vi "通道设置.vi"(0 "Channel (0: Channel 1)":u16(ring) items=["Channel 1", "Channel 2", "Channel 3", "Channel 4", "Math", "Reference 1", "Reference 2", "Reference 3", "Reference 4", "Bus 1", "Bus 2"], 1 "范围 (10.0 V)":dbl=10.0, 2 "VISA resource name":refnum<visa-resource-name>, 3 "带宽 (0: FULL)":u16(ring) items=["FULL", "250 MHz", "150 MHz", "20 MHz"], 5 "偏置 (0.0 V)":dbl, 9 "衰减 (1)":dbl=1.0, 11 "耦合(1: DC)":u16(ring)=1 items=["AC", "DC", "Ground"], 12 "输入阻抗 (0: 1M ohm)":u16(ring) items=["1M", "75", "50"], 13 "error in (no error)":errorcluster, 14 "通道使能 (T: Enable)":bool=TRUE) -> (4 "VISA resource name out":refnum<visa-resource-name>, 15 "error out":errorcluster)   [LabVIEW 2018]
uses:
  Tektronix DPO MSO 2000 4000 Series/Tektronix DPO MSO 2000 4000 Series.lvlib
panel:
  out "写入缓冲区":string
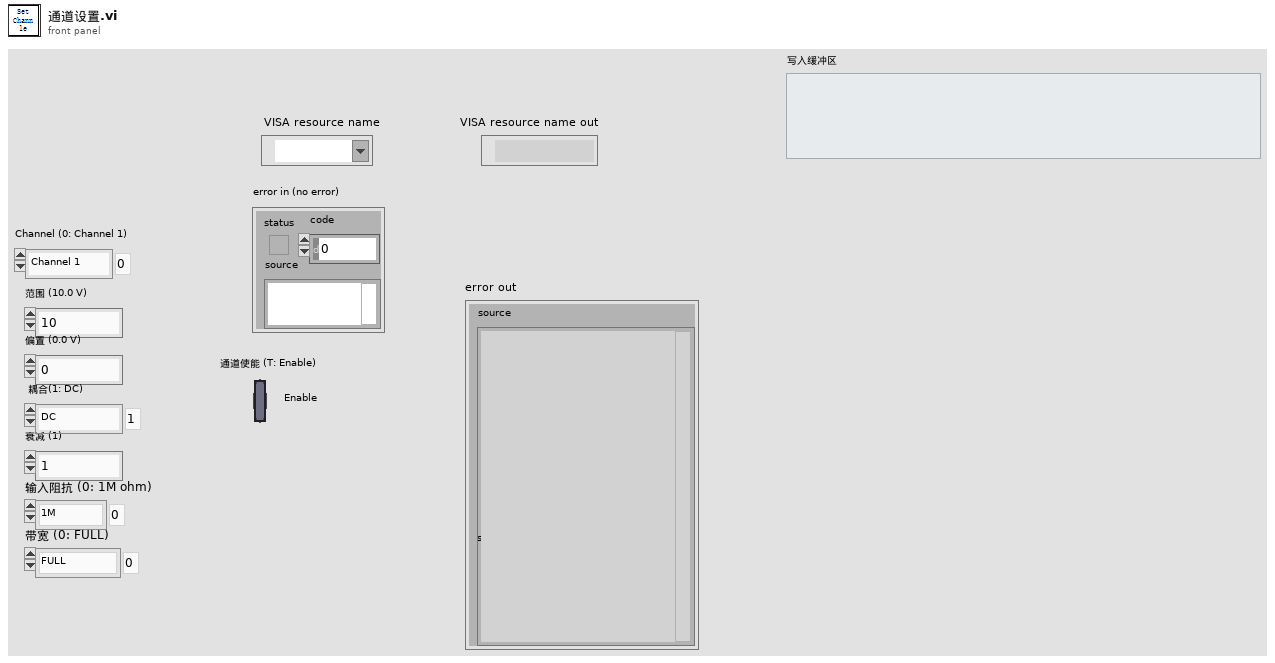
[diagram p1: front panel]
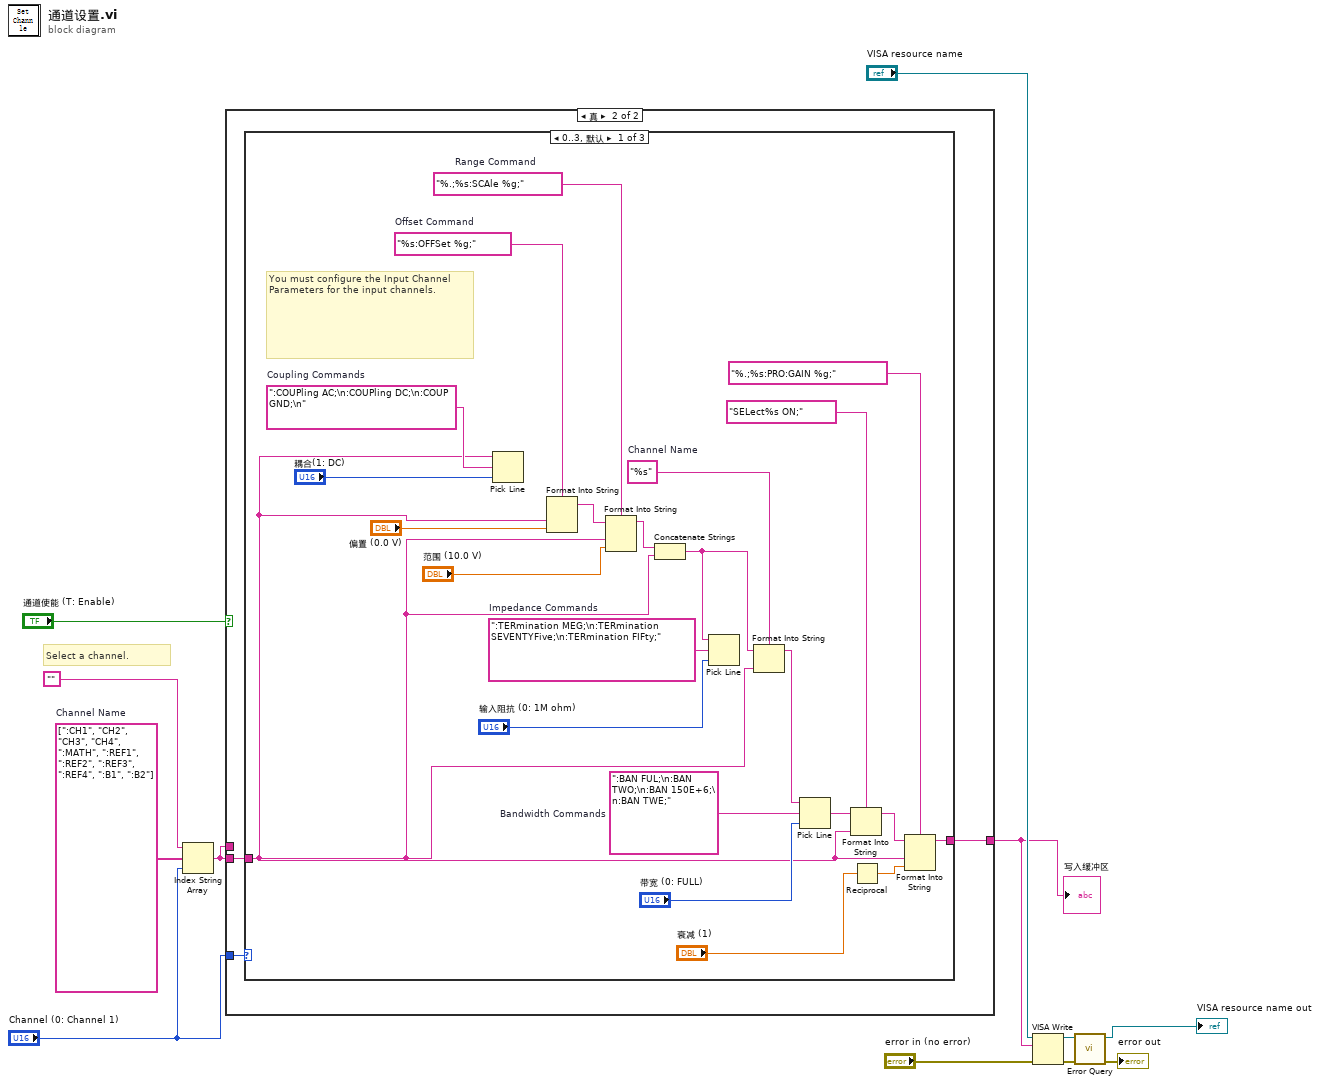
[diagram p0: block diagram]
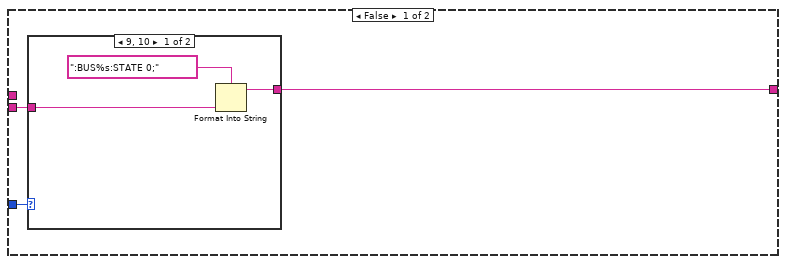
[diagram p2: hidden frame]
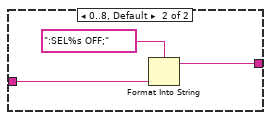
[diagram p3: hidden frame]
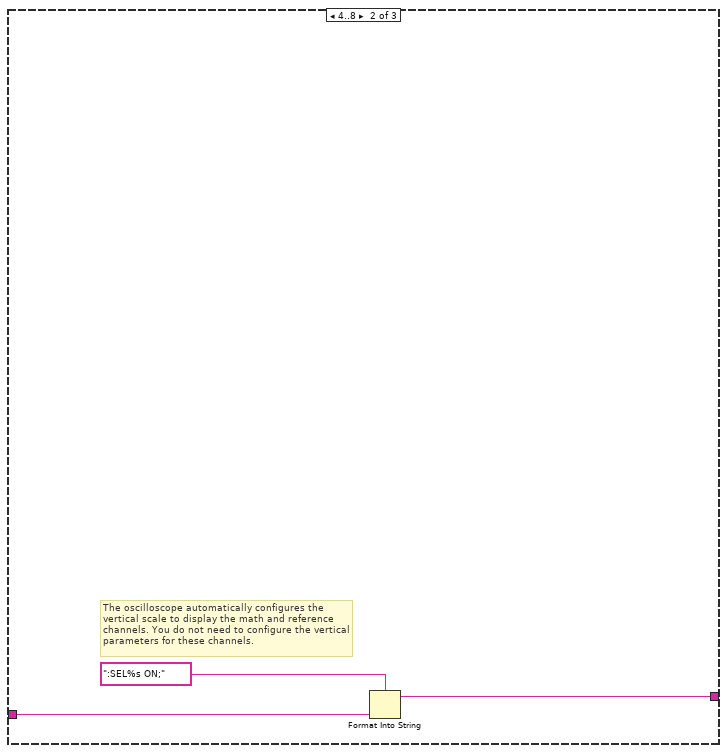
[diagram p4: hidden frame]
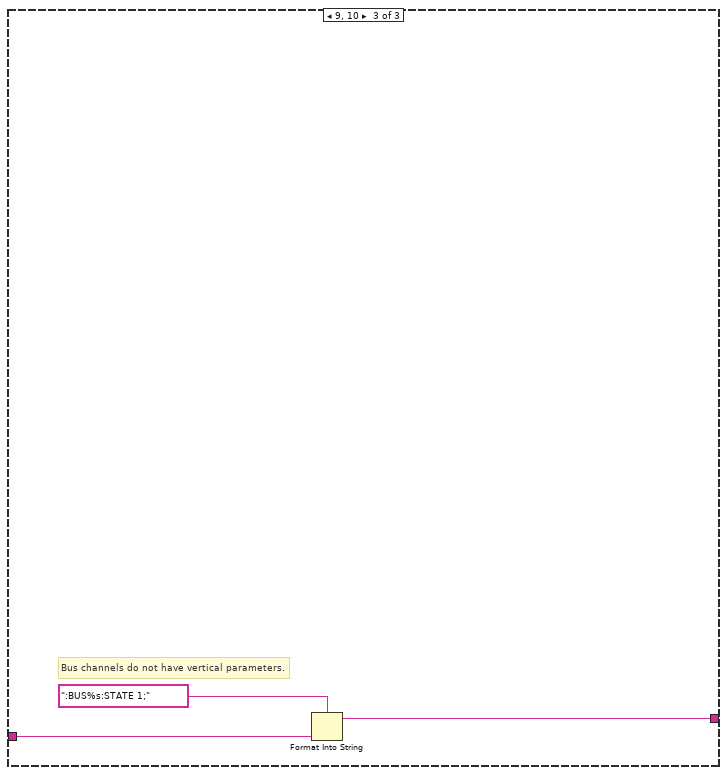
[diagram p5: hidden frame]
diagram:
  w11 = string[] [":CH1", "CH2", "CH3", "CH4", ":MATH", ":REF1", ":REF2", ":REF3", ":REF4", ":B1", ":B2"]  # Channel Name
  # "Select a channel."
  n1 = Index String Array(1:"Channel (0: Channel 1)", 2:w11, 3:"") -> (0:w8:string)
  n2 = case shown="真" "通道使能 (T: Enable)" {
    tunnel: "Channel (0: Channel 1)" -> [w15 w24]
    tunnel: [w14 w23] -> w1
    tunnel: w8 -> [_ _]
    tunnel: w8 -> [w13 w22]
    frame False {
      n3 = case shown="9, 10" w15 {
        tunnel: [w17 w20] -> w14
        tunnel: w13 -> [w16 w19]
        frame 9, 10 {
          n4 = Format Into String(format string=":BUS%s:STATE 0;", w16) -> (resulting string=w17:string)  [unwired: 2 in, 1 out]
        }
        frame 0..8, Default {
          n5 = Format Into String(format string=":SEL%s OFF;", w19) -> (resulting string=w20:string)  [unwired: 2 in, 1 out]
        }
      }
    }
    frame True {
      n6 = case shown="0..3, 默认" w24 {
        tunnel: [w31 w49 w52] -> w23
        tunnel: w22 -> [w26 w48 w51]
        frame 0..3, Default {
          w37 = ":BAN FUL;\n:BAN TWO;\n:BAN 150E+6;\n:BAN TWE;"  # Bandwidth Commands
          w39 = "%s"  # Channel Name
          w40 = ":TERmination MEG;\n:TERmination SEVENTYFive;\n:TERmination FIFty;"  # Impedance Commands
          w43 = "%.;%s:SCAle %g;"  # Range Command
          w45 = "%s:OFFSet %g;"  # Offset Command
          w47 = ":COUPling AC;\n:COUPling DC;\n:COUP GND;\n"  # Coupling Commands
          # "You must configure the Input Channel\nParameters for the input channels."
          n7 = Pick Line(string ("")=w26, multi-line string=w47, line index="耦合(1: DC)") -> ()  [unwired: 1 out]
          n8 = Format Into String(format string=w45, w26, "偏置 (0.0 V)") -> (resulting string=w42:string)  [unwired: 2 in, 1 out]
          n9 = Format Into String(format string=w43, initial string=w42, w26, "范围 (10.0 V)") -> (resulting string=w27:string)  [unwired: 1 in, 1 out]
          n10 = Concatenate Strings(w27, w26) -> (w25:string)
          n11 = Pick Line(string ("")=w25, multi-line string=w40, line index="输入阻抗 (0: 1M ohm)") -> ()  [unwired: 1 out]
          n12 = Format Into String(format string=w39, initial string=w25, w26) -> (resulting string=w38:string)  [unwired: 1 in, 1 out]
          n13 = Pick Line(string ("")=w38, multi-line string=w37, line index="带宽 (0: FULL)") -> (output string=w34:string)
          n14 = Format Into String(format string="SELect%s ON;", initial string=w34, w26) -> (resulting string=w33:string)  [unwired: 1 in, 1 out]
          n15 = Reciprocal(x="衰减 (1)") -> (1/x=w30:dbl)
          n16 = Format Into String(format string="%.;%s:PRO:GAIN %g;", initial string=w33, w26, w30) -> (resulting string=w31:string)  [unwired: 1 in, 1 out]
        }
        frame 4..8 {
          # "The oscilloscope automatically configures the vertical scale to display the math and reference channels. You do not need to configure the vertical parameters for these channels."
          n17 = Format Into String(format string=":SEL%s ON;", w48) -> (resulting string=w49:string)  [unwired: 2 in, 1 out]
        }
        frame 9, 10 {
          # "Bus channels do not have vertical parameters."
          n18 = Format Into String(format string=":BUS%s:STATE 1;", w51) -> (resulting string=w52:string)  [unwired: 2 in, 1 out]
        }
      }
    }
  }
  "写入缓冲区" <- w1
  n19 = VISA Write(VISA resource name="VISA resource name", write buffer=w1, error in (no error)="error in (no error)") -> (VISA resource name out=w5:refnum<visa-resource-name>, error out=w4:errorcluster)  [unwired: 1 out]
  n20 = call "Error Query.vi"("error in (no error)"=w4, "VISA resource name"=w5) -> ("error out"=→"error out":errorcluster, "VISA resource name out"=→"VISA resource name out":refnum<visa-resource-name>)  [unwired: 6 in, 2 out]
